vi "GetHisto.vi"() -> ()   [LabVIEW 2014]
uses:
  <vilib>/Analysis/NI_AALBase.lvlib
  <vilib>/Analysis/NI_AALPro.lvlib
panel:
  out "appended array":dbl[](array[numeric])
  out "x-y":u32
  out "Histogram Graph 2":T1(graph)
  out "Numeric":i32
  out "Histogram Graph":T1(graph)
  in  "VISA resource name":refnum<visa-resource-name>
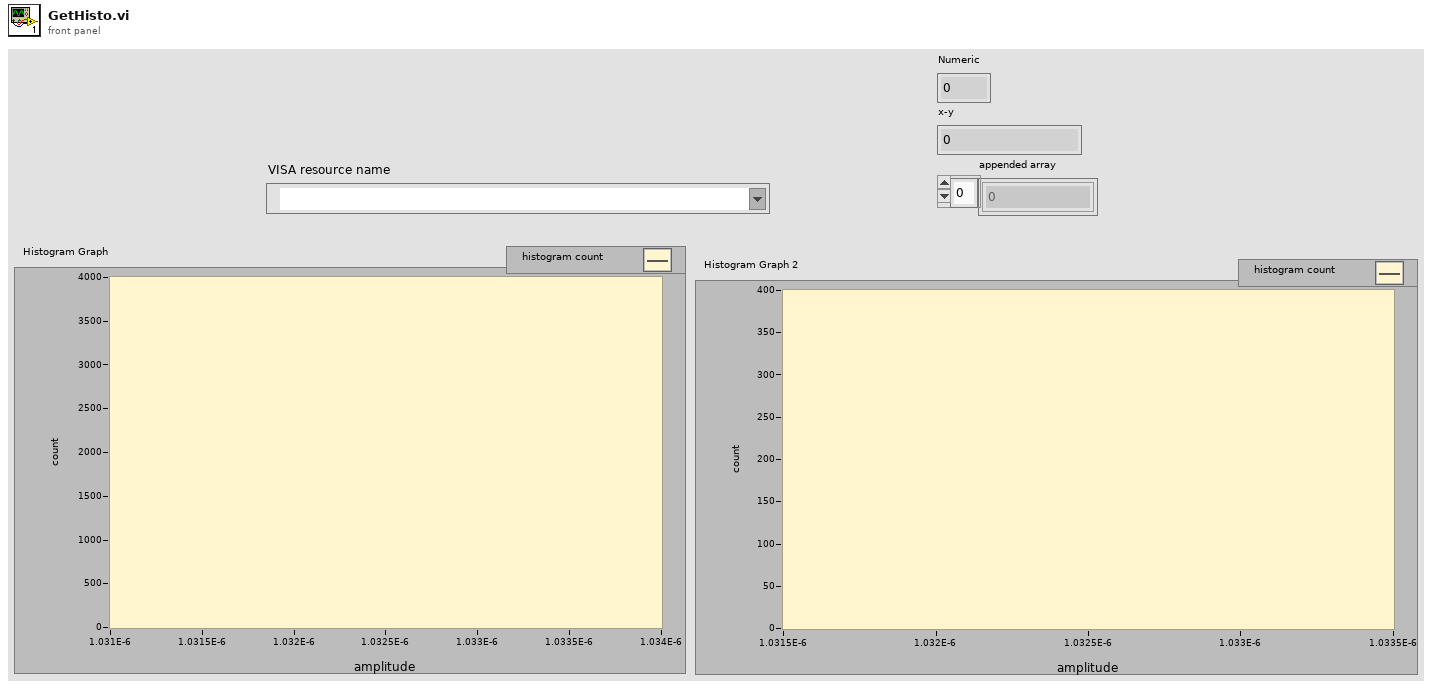
[diagram p1: front panel]
types:
  T1 = cluster{"X Values":dbl[], "Histogram: h(x)":i32[]}
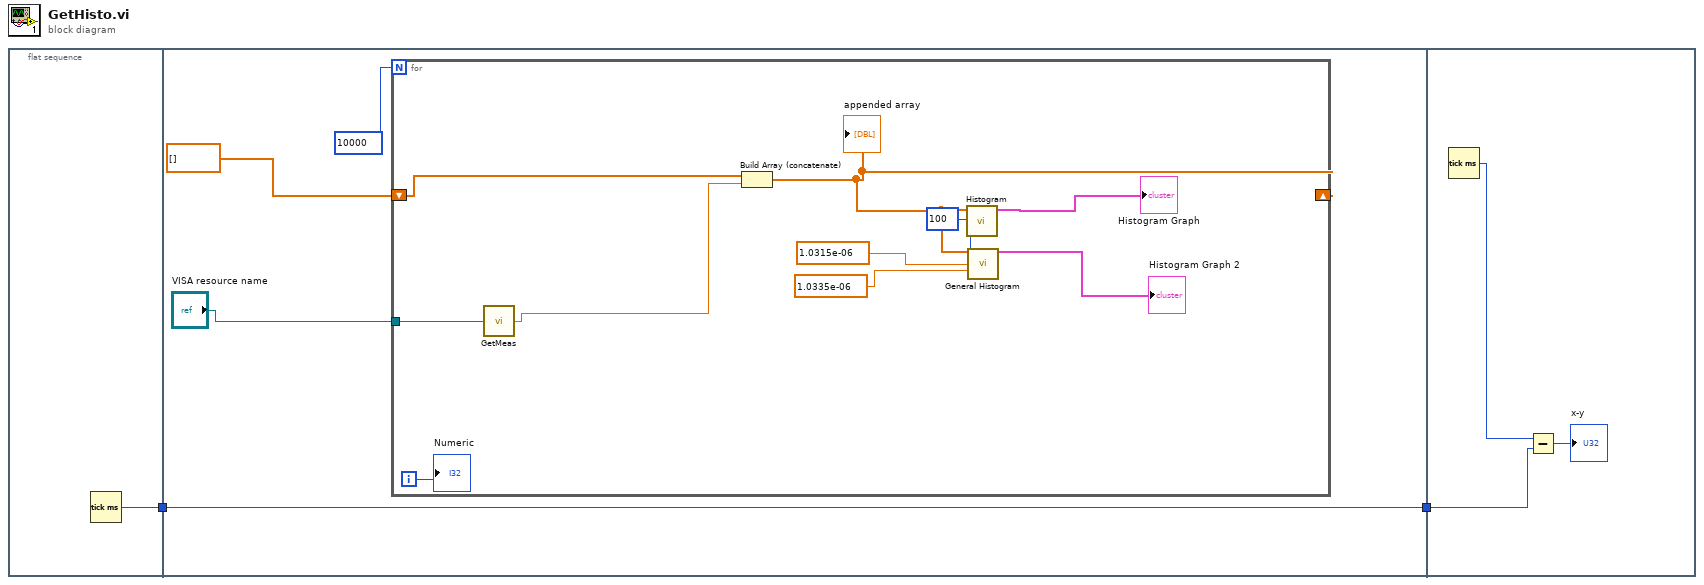
[diagram p0: block diagram]
diagram:
  n1 = flat-sequence {
    tunnel: [w3] -> w1
    tunnel: [w4] -> w2
    tunnel: w1 -> [w4]
    tunnel: w2 -> [w19]
    frame #0 {
      n2 = Tick Count (ms)() -> (millisecond timer value=w3:u32)
    }
    frame #1 {
      n3 = for {
        N: 10000 -> [_]
        tunnel: "VISA resource name" -> [w9]
        shift-right: [w10] -> _
        shift-left: dbl[] [] -> [w11]
        i -> [w17]
        n4 = call "GetMeas.vi"("VISA resource name"=w9) -> ("Numeric Control"=w8:dbl)
        n5 = Build Array (concatenate)(w11, w8) -> (w10:dbl[])
        "appended array" <- w10
        n6 = call <vilib>:"Histogram.vi"("X"=w10) -> ("Histogram Graph"=→"Histogram Graph":T1)  [unwired: 7 in, 3 out]
        n7 = call <vilib>:"General Histogram.vi"("X"=w10, "max"=1.0315e-06, "min"=1.0335e-06, "# bins"=100) -> ("Histogram Graph"=→"Histogram Graph 2":T1)  [unwired: 7 in, 4 out]
        "Numeric" <- w17
      }
    }
    frame #2 {
      n8 = Tick Count (ms)() -> (millisecond timer value=w20:u32)
      n9 = Subtract(x=w20, y=w19) -> (x-y=→"x-y":u32)
    }
  }
